vi "SplitDataSetXY.vi"(7 "%SplitTrain":i32=80 min=1 max=100 step=1 format="%.0f %", 8 "error in (no error)":errorcluster, 10 "Y":dbl[][](array[numeric]), 11 "X":dbl[][](array[numeric])) -> (0 "error out":errorcluster, 3 "Split":T1)   [LabVIEW 2020]
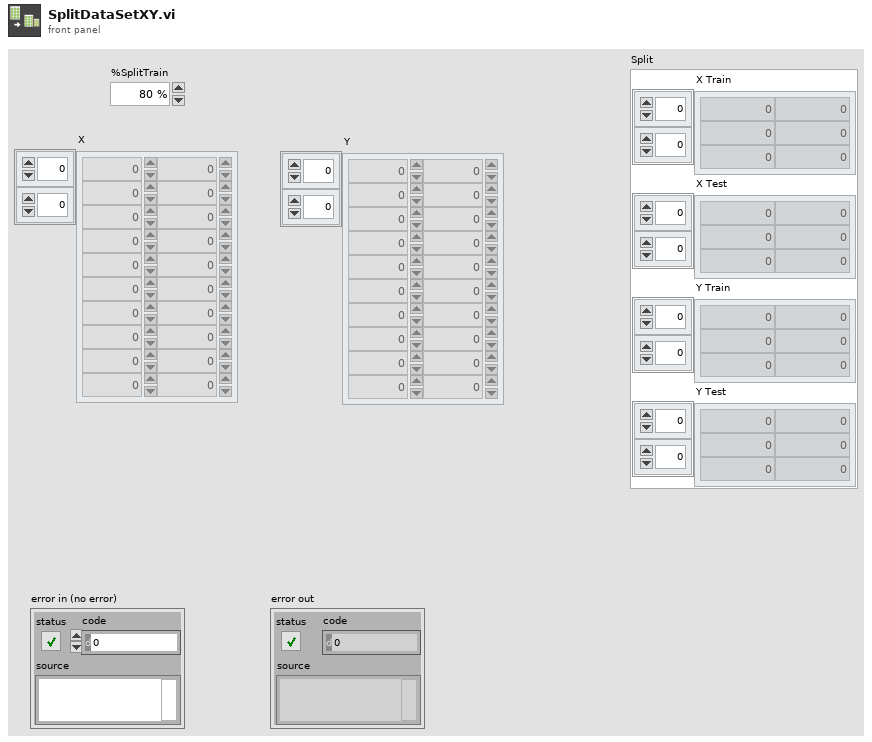
[diagram p1: front panel]
types:
  T1 = cluster{"X Train":dbl[][], "X Test":dbl[][], "Y Train":dbl[][], "Y Test":dbl[][]}
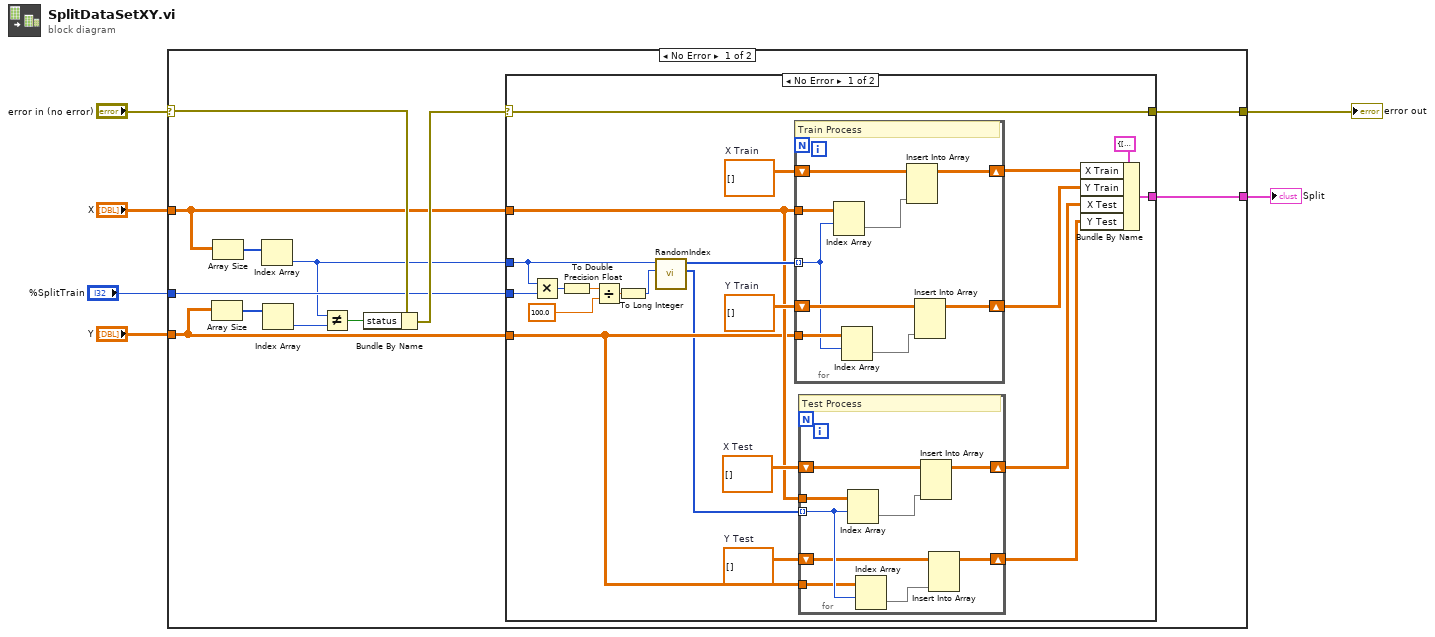
[diagram p0: block diagram]
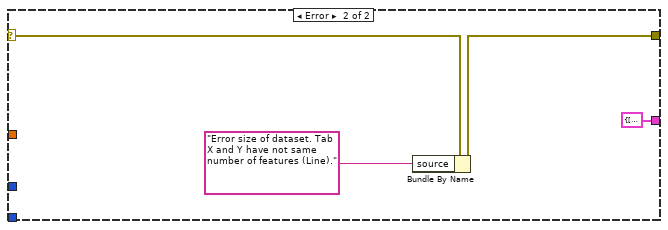
[diagram p2: hidden frame]
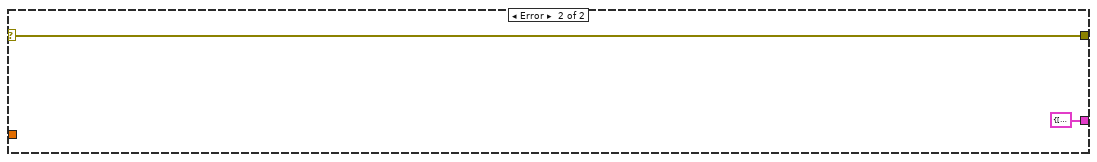
[diagram p3: hidden frame]
diagram:
  n1 = case shown="No Error" "error in (no error)" {
    selector: "error in (no error)" -> [w12 w64]
    tunnel: [w18 w64] -> w6
    tunnel: "Y" -> [w11 _]
    tunnel: "X" -> [w10 _]
    tunnel: "%SplitTrain" -> [w9 _]
    tunnel: [w7 T1 {"X Train"=[], "X Test"=[], "Y Train"=[], "Y Test"=[]} ("Split")] -> w1
    frame No Error {
      n2 = Array Size(array=w11) -> (size(s)=w16:i32[])
      n3 = Array Size(array=w10) -> (size(s)=w15:i32[])
      n4 = Index Array(array=w15) -> (element=w8:i32)  [unwired: 1 in]
      n5 = Index Array(array=w16) -> (element=w17:i32)  [unwired: 1 in]
      n6 = Not Equal?(x=w8, y=w17) -> (x != y?=w13:bool)
      n7 = Bundle By Name(cluster=w12, "status"=w13) -> (w14:errorcluster)
      n8 = case shown="No Error" w14 {
        selector: w14 -> [w40 w62]
        tunnel: [w40 w61] -> w18
        tunnel: w10 -> [w25 _]
        tunnel: w11 -> [w22 _]
        tunnel: w9 -> [w33 _]
        tunnel: w8 -> [w34 _]
        tunnel: [w19 T1 {"X Train"=[], "X Test"=[], "Y Train"=[], "Y Test"=[]} ("Split")] -> w7
        frame No Error {
          w26 = dbl[][] []  # Y Test
          w27 = dbl[][] []  # X Test
          w36 = dbl[][] []  # Y Train
          w39 = dbl[][] []  # X Train
          n9 = Multiply(x=w34, y=w33) -> (x*y=w32:i32)
          n10 = To Double Precision Float(number=w32) -> (double precision float=w30:dbl)
          n11 = Divide(x=w30, y=100.0) -> (x/y=w29:dbl)
          n12 = To Long Integer(number=w29) -> (32bit integer=w28:i32)
          n13 = call "RandomIndex.vi"("Nbre de valeur"=w28, "Taille du tab"=w34) -> ("RandomComplementaryIndex"=w21:i32[], "RandomIndex"=w37:i32[])  [unwired: 8 in]
          n14 = for {
            tunnel: w25 -> [w56]
            shift-right: [w57] -> w38
            shift-left: w39 -> [w58]
            tunnel: w37 -> [w50] mode=indexing
            shift-right: [w52] -> w35
            shift-left: w36 -> [w53]
            tunnel: w22 -> [w51]
            # "Train Process"
            n15 = Index Array(array=w56, index (row)=w50) -> (element=w55:dbl[])  [unwired: 1 in]
            n16 = Index Array(array=w51, index (row)=w50) -> (element=w54:dbl[])  [unwired: 1 in]
            n17 = Insert Into Array(array=w58, new element=w55) -> (w57:dbl[][])  [unwired: 2 in]
            n18 = Insert Into Array(array=w53, new element=w54) -> (w52:dbl[][])  [unwired: 2 in]
          }
          n19 = for {
            tunnel: w25 -> [w45]
            shift-right: [w46] -> w24
            shift-left: w27 -> [w47]
            shift-right: [w41] -> w23
            shift-left: w26 -> [w43]
            tunnel: w22 -> [w42]
            tunnel: w21 -> [w44] mode=indexing
            # "Test Process"
            n20 = Index Array(array=w45, index (row)=w44) -> (element=w49:dbl[])  [unwired: 1 in]
            n21 = Index Array(array=w42, index (row)=w44) -> (element=w48:dbl[])  [unwired: 1 in]
            n22 = Insert Into Array(array=w47, new element=w49) -> (w46:dbl[][])  [unwired: 2 in]
            n23 = Insert Into Array(array=w43, new element=w48) -> (w41:dbl[][])  [unwired: 2 in]
          }
          n24 = Bundle By Name(cluster=T1 {"X Train"=[], "X Test"=[], "Y Train"=[], "Y Test"=[]} ("Split"), "X Train"=w38, "Y Train"=w35, "X Test"=w24, "Y Test"=w23) -> (w19:T1)
        }
        frame Error {
          n25 = Bundle By Name(cluster=w62, "source"="Error size of dataset. Tab X and Y have not same number of features (Line).") -> (w61:errorcluster)
        }
      }
    }
    frame Error {
    }
  }
  "error out" <- w6
  "Split" <- w1
